vi "STATION.vi"(6 "station":T4, 8 "error_in":errorcluster, 11 "all_config_info":T1) -> (0 "error_out":errorcluster)   [LabVIEW 2020]
uses:
  station.ctl
  ini/typedef/PROXY_all_config_info.ctl
  ini/typedef/PROXY_main_ini_file.ctl
  queues/typedef/PROXY_queue_refnums.ctl
  queues/typedef/STATION_queue_element.ctl
  ST_SQL_sequence_state.ctl
  ST_TCP_sequence_state.ctl
  FGV/DIAGNOSTICS_records_display/FGV_PROXY_DIAGNOSTICS_records_display.ctl
  MAIN/DIAGNOSTICS/PROXY_SQL_connection_status.ctl
  FGV/SQL_part_ID_buffer/FGV_SQL_part_ID_buffer.ctl
  FGV/SQL_pinion_ID_buffer/FGV_SQL_pinion_ID_buffer.ctl
  FGV/connection_references/FGV_PROXY_connection_references.ctl
  FGV/DIAGNOSTICS_message_history_buffer/FGV_PROXY_DIAGNOSTICS_message_history_buffer.ctl
  FGV/error_buffer/FGV_PROXY_error_buffer.ctl
  <vilib>/addons/database/Connection.llb/Conn ObjectReference.ctl
  _misc/PLC_connection_status.ctl
  <vilib>/addons/database/Connection.llb/DB Tools Open Connec (String).vi
  _misc/byte_array_parser/to_U16.vi
  _misc/byte_array_parser/to_string.vi
  _misc/byte_array_parser/to_U8.vi
  _misc/AULocalize/SubVIs/Get Localized Phrase Compact Interface 0D.vi
  <vilib>/addons/database/NI_Database_API.lvlib
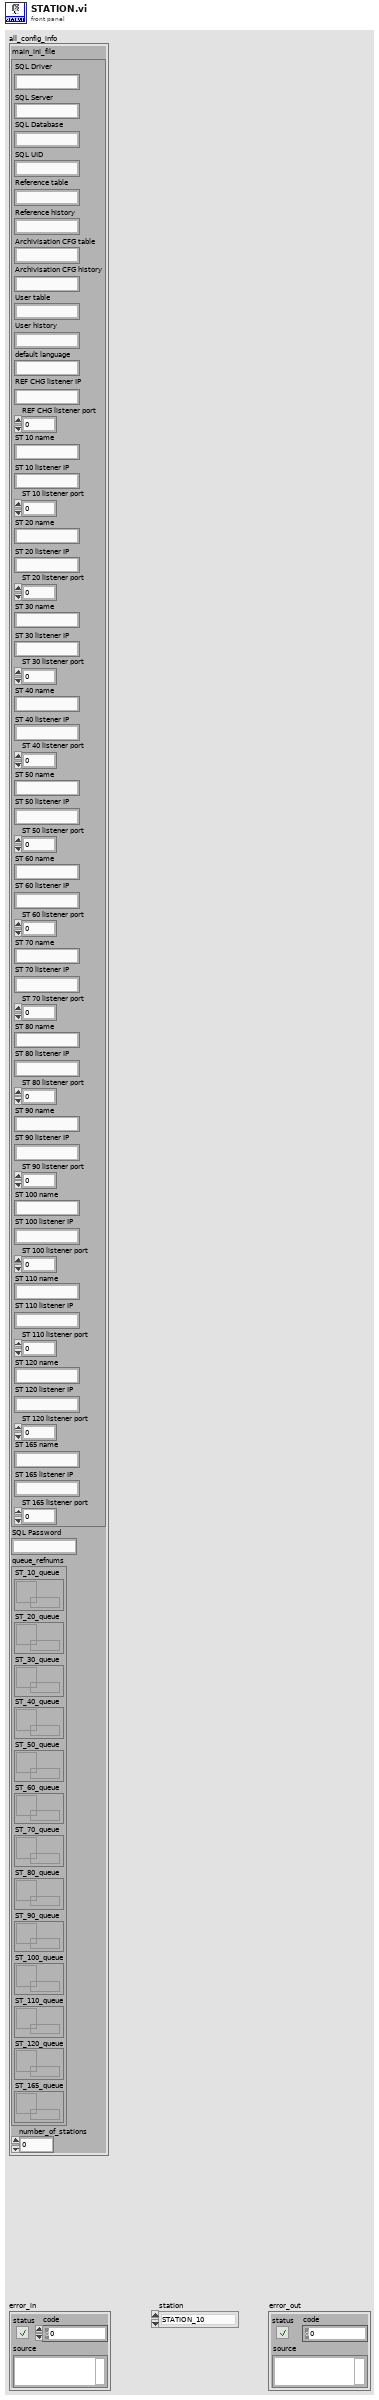
[diagram p1: front panel]
types:
  T1 = typedef "PROXY_all_config_info.ctl" = cluster{"main_ini_file":T2, "SQL Password":string, "queue_refnums":T3, "number_of_stations":i32}
  T2 = typedef "PROXY_main_ini_file.ctl" = cluster{"SQL Driver":string, "SQL Server":string, "SQL Database":string, "SQL UID":string, "Reference table":string, "Reference history":string, "Archivisation CFG table":string, "Archivisation CFG history":string, "User table":string, "User history":string, "default language":string, "REF CHG listener IP":string, "REF CHG listener port":u16, "ST 10 name":string, "ST 10 listener IP":string, "ST 10 listener port":u16, "ST 20 name":string, "ST 20 listener IP":string, "ST 20 listener port":u16, "ST 30 name":string, "ST 30 listener IP":string, "ST 30 listener port":u16, "ST 40 name":string, "ST 40 listener IP":string, "ST 40 listener port":u16, "ST 50 name":string, "ST 50 listener IP":string, "ST 50 listener port":u16, "ST 60 name":string, "ST 60 listener IP":string, "ST 60 listener port":u16, "ST 70 name":string, "ST 70 listener IP":string, "ST 70 listener port":u16, "ST 80 name":string, "ST 80 listener IP":string, "ST 80 listener port":u16, "ST 90 name":string, "ST 90 listener IP":string, "ST 90 listener port":u16, "ST 100 name":string, "ST 100 listener IP":string, "ST 100 listener port":u16, "ST 110 name":string, "ST 110 listener IP":string, "ST 110 listener port":u16, "ST 120 name":string, "ST 120 listener IP":string, "ST 120 listener port":u16, "ST 165 name":string, "ST 165 listener IP":string, "ST 165 listener port":u16}
  T3 = typedef "PROXY_queue_refnums.ctl" = cluster{"ST_10_queue":refnum<queue>, "ST_20_queue":refnum<queue>, "ST_30_queue":refnum<queue>, "ST_40_queue":refnum<queue>, "ST_50_queue":refnum<queue>, "ST_60_queue":refnum<queue>, "ST_70_queue":refnum<queue>, "ST_80_queue":refnum<queue>, "ST_90_queue":refnum<queue>, "ST_100_queue":refnum<queue>, "ST_110_queue":refnum<queue>, "ST_120_queue":refnum<queue>, "ST_165_queue":refnum<queue>}
  T4 = typedef "station.ctl" = enum16{"STATION_10", "STATION_20", "STATION_30", "STATION_40", "STATION_50", "STATION_60", "STATION_70", "STATION_80", "STATION_90", "STATION_100", "STATION_110", "STATION_120", "STATION_165", "MAIN"}
  T5 = typedef "ST_TCP_sequence_state.ctl" = enum16{"initialize", "wait_for_connection", "handle_message", "error", "stop"}
  T6 = typedef "ST_SQL_sequence_state.ctl" = enum16{"initialize", "get_next_state", "send_to_SQL", "send_to_PLC", "error", "stop"}
  T7 = typedef "FGV_PROXY_connection_references.ctl" = enum16{"initialize", "set_listener_ID", "set_connection_ID", "get", "KILL_ALL_CONNECTIONS", "killed?"}
  T8 = typedef "PLC_connection_status.ctl" = enum16{"Connected", "Waiting", "Error", "-"}
  T9 = typedef "FGV_PROXY_DIAGNOSTICS_records_display.ctl" = enum16{"initialize", "set_PLC_IP", "set_PLC_Port", "set_PLC_connection_status", "set_SQL_connection_status", "get_all_info"}
  T10 = enum16{"Standard", "Buffered", "CRLF", "Immediate"}
  T11 = typedef "STATION_queue_element.ctl" = cluster{"state":T6, "variable":variant}
  T12 = typedef "FGV_PROXY_DIAGNOSTICS_message_history_buffer.ctl" = enum16{"initialize", "add_TCP_PLC_to_PC", "add_TCP_PC_to_PLC", "add_SQL_PC_to_DB", "add_SQL_transaction", "add_SQL_DB_to_PC", "get_station", "get_all", "clear_station", "clear_all", "save_log"}
  T13 = typedef "FGV_PROXY_error_buffer.ctl" = enum16{"initialize", "clear", "display", "get_status"}
  T14 = typedef "PROXY_SQL_connection_status.ctl" = enum16{"Connected", "Waiting", "Error", "-"}
  T15 = typedef "FGV_SQL_part_ID_buffer.ctl" = enum16{"initialize", "buffer_serial_ID", "get_ID_for_name"}
  T16 = typedef "FGV_SQL_pinion_ID_buffer.ctl" = enum16{"initialize", "buffer_pinion_ID", "buffer_pinion_ID_SQL", "get_ID_for_name"}
  T17 = typedef "NI_Database_API.lvlib/Conn ObjectReference.ctl" = refnum<k1>
  T18 = typedef "SQL_statuses.ctl" = enum16{"OK", "PART_IN_OPERATION", "PART_DOES_NOT_EXIST", "OPERATION_DOES_NOT_EXIST", "OPERATOR_DOES_NOT_EXIST", "PART_NOT_IN_OPERATION"}
  T19 = typedef "ST_results_info.ctl" = cluster{"INT_number":i32, "REAL_number":i32, "STRING_number":i32, "STRING_length":i32, "BATCH_number":i32, "BATCH_length":i32, "INT_array":i16[], "REAL_array":sgl[], "STRING_array":string[], "BATCH_array":string[]}
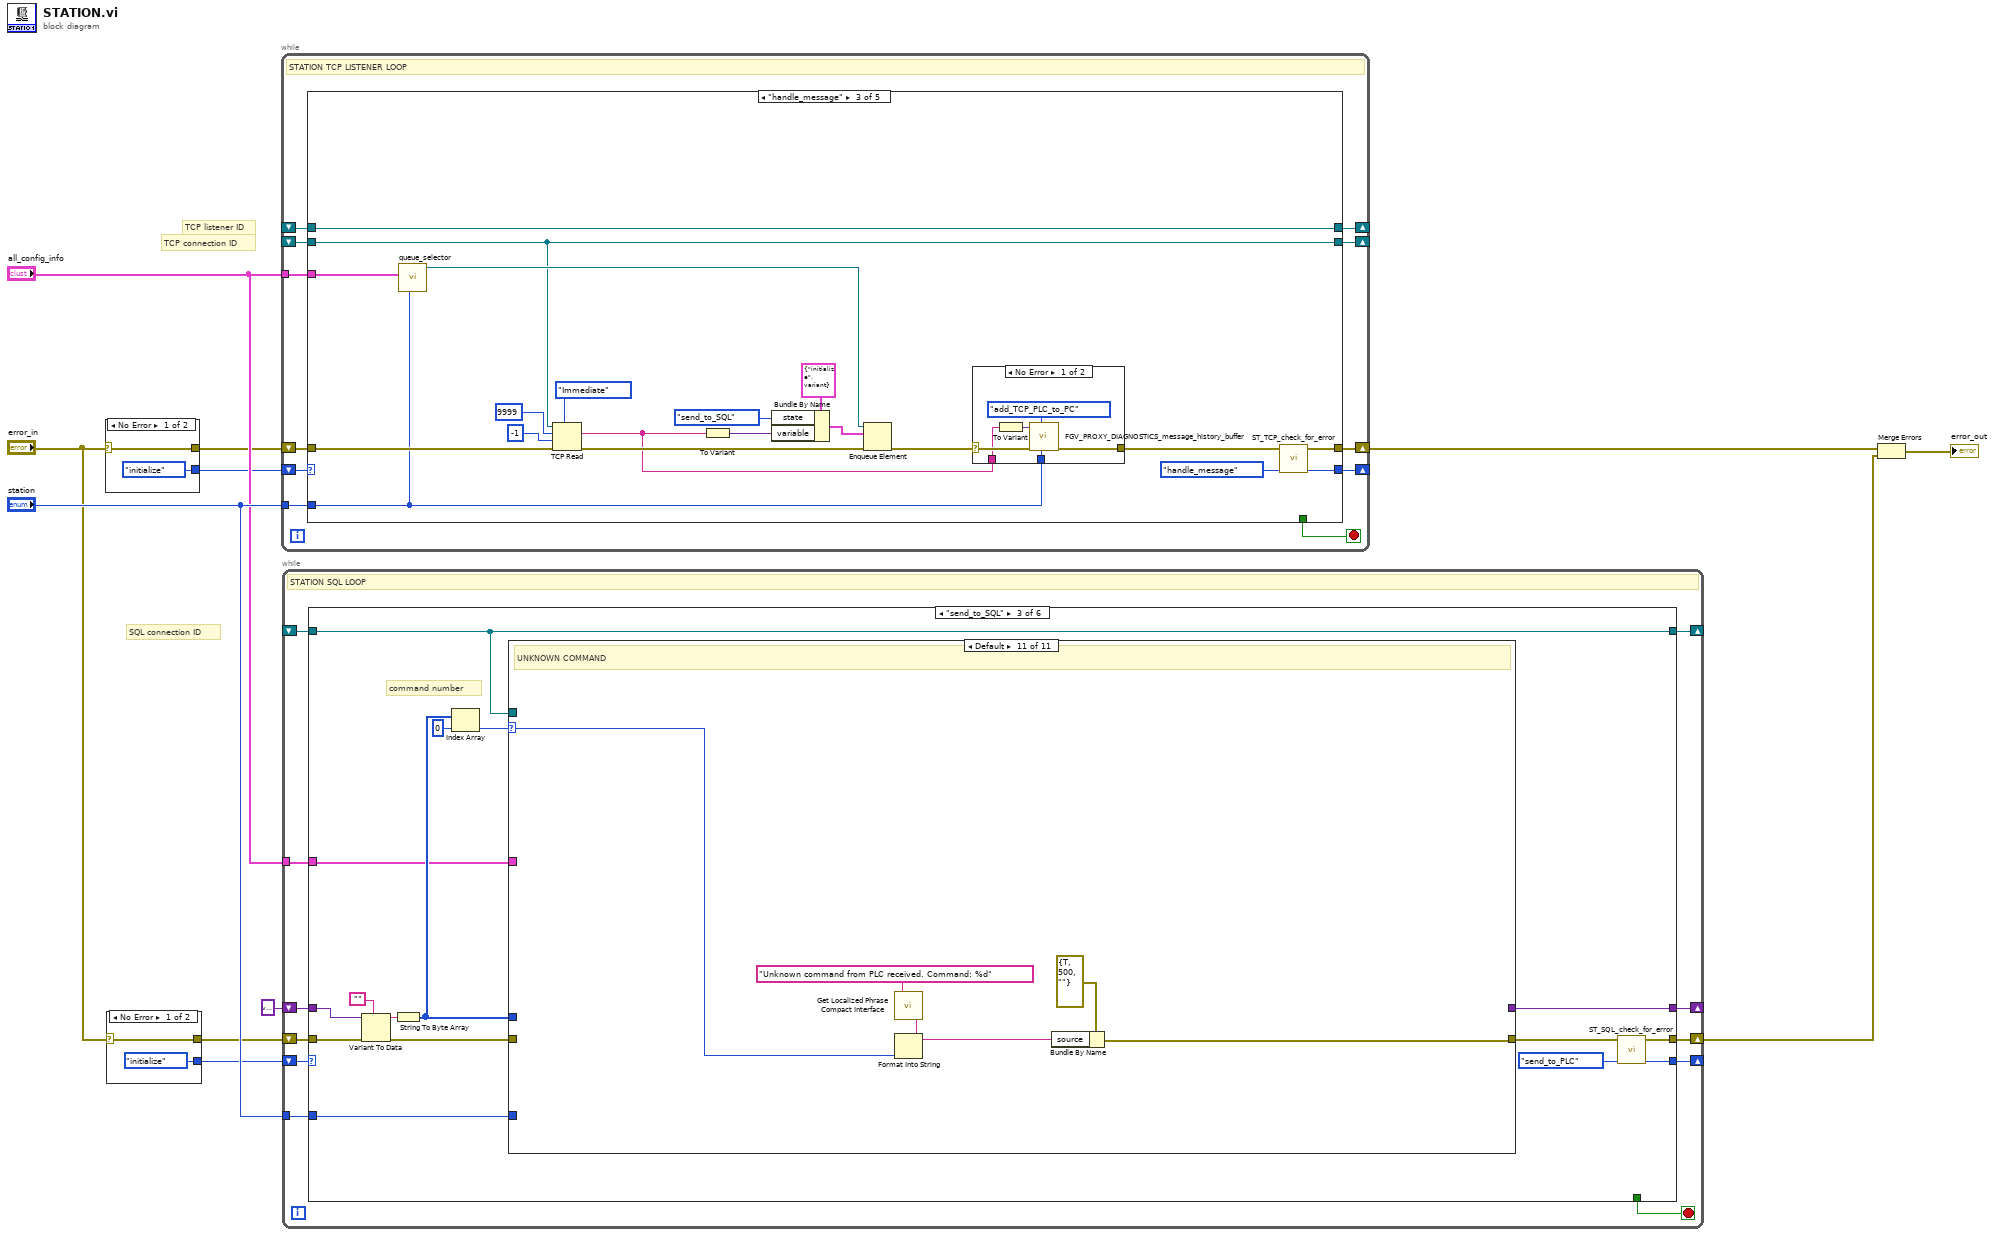
[diagram p0: block diagram]
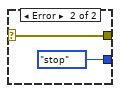
[diagram p2: hidden frame]
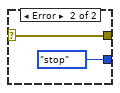
[diagram p3: hidden frame]
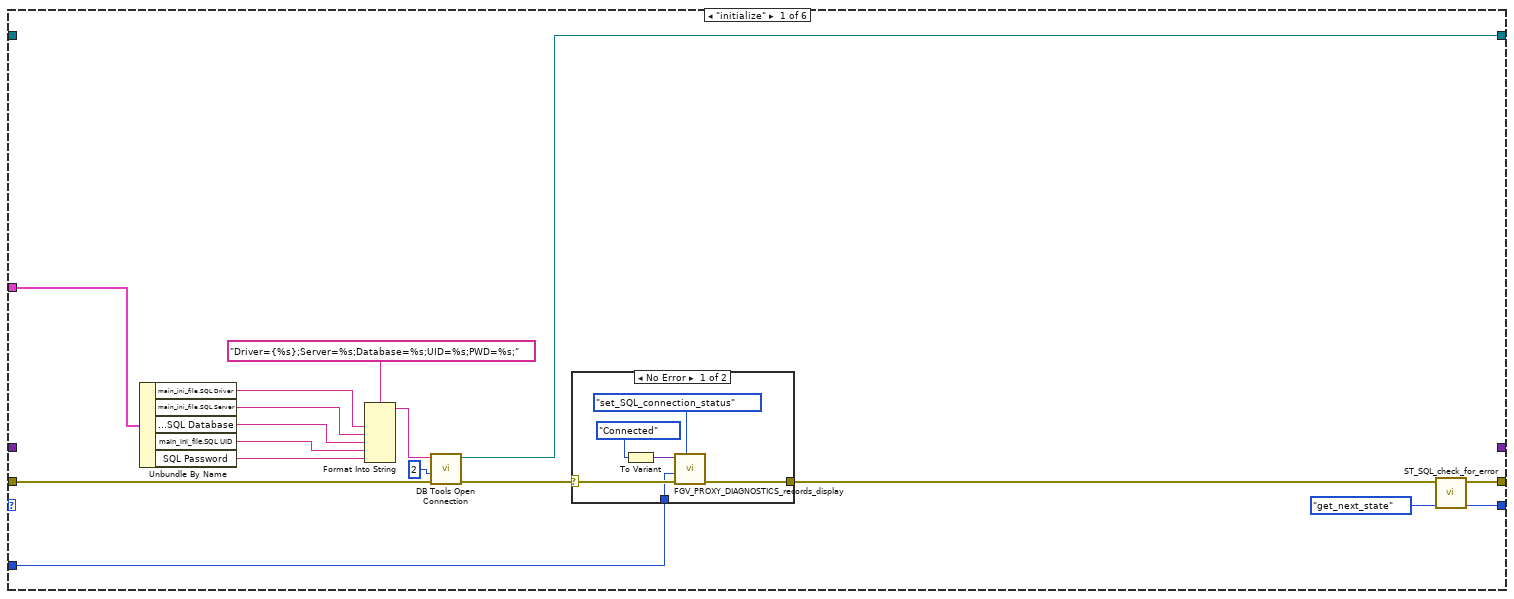
[diagram p4: hidden frame]
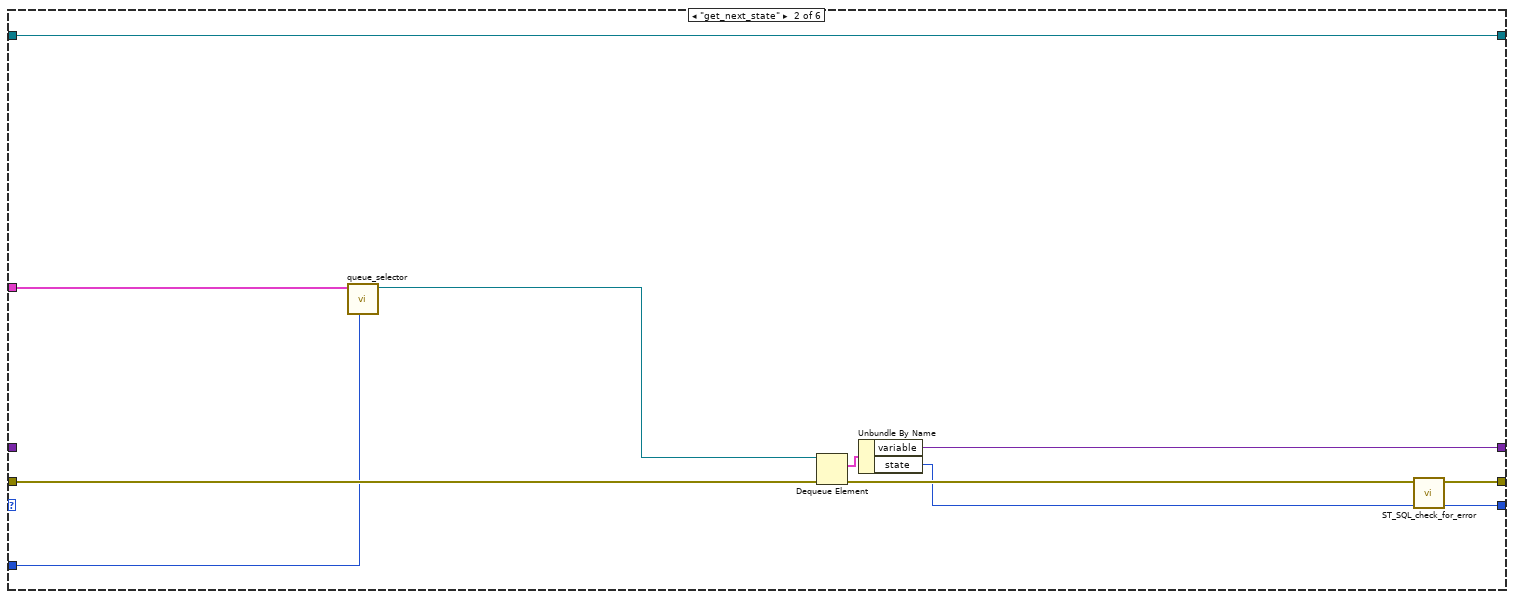
[diagram p6: hidden frame]
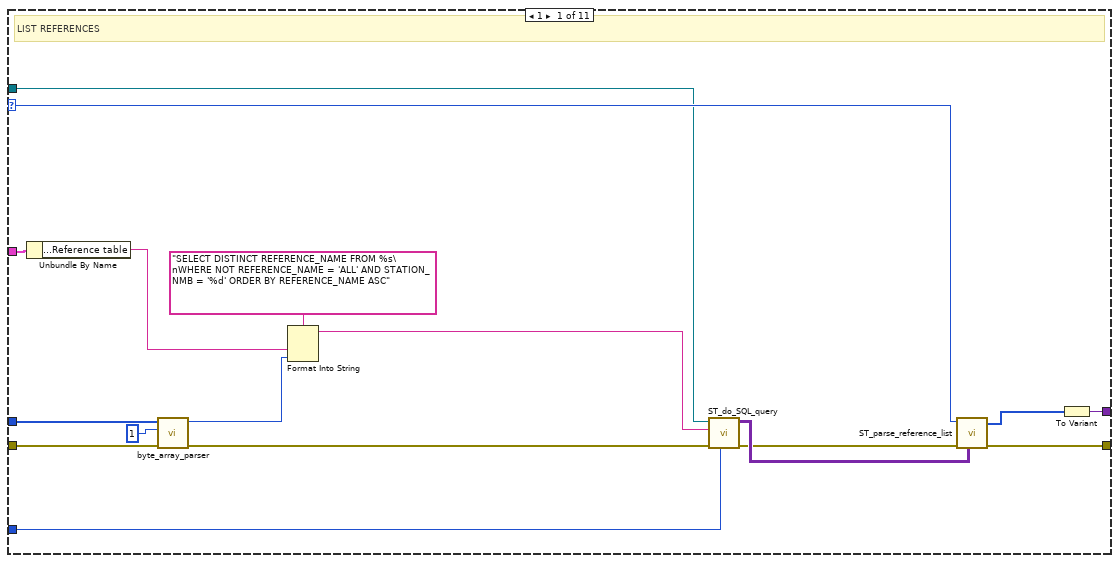
[diagram p7: hidden frame]
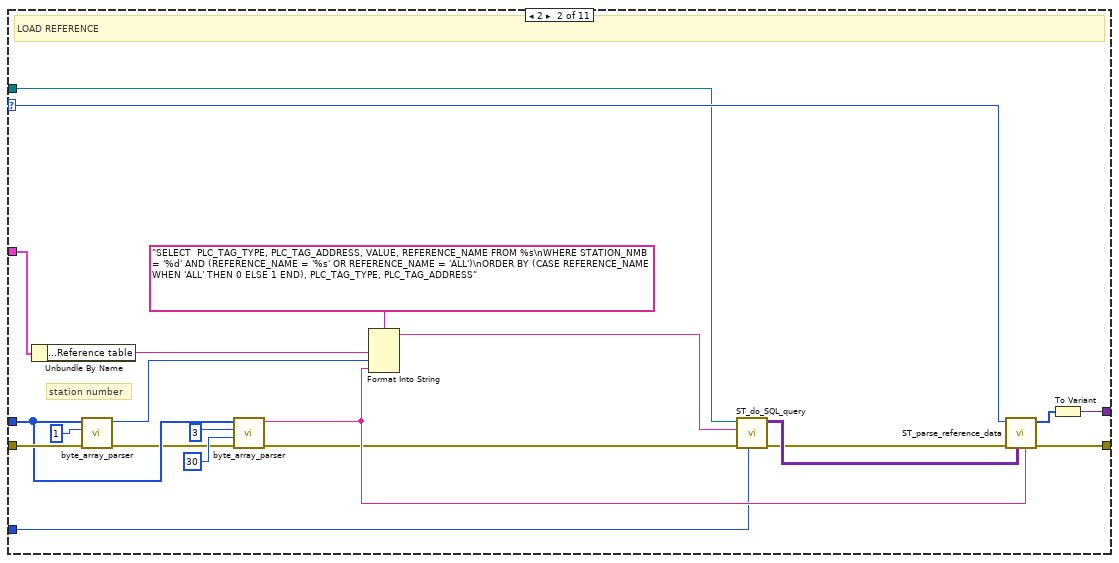
[diagram p8: hidden frame]
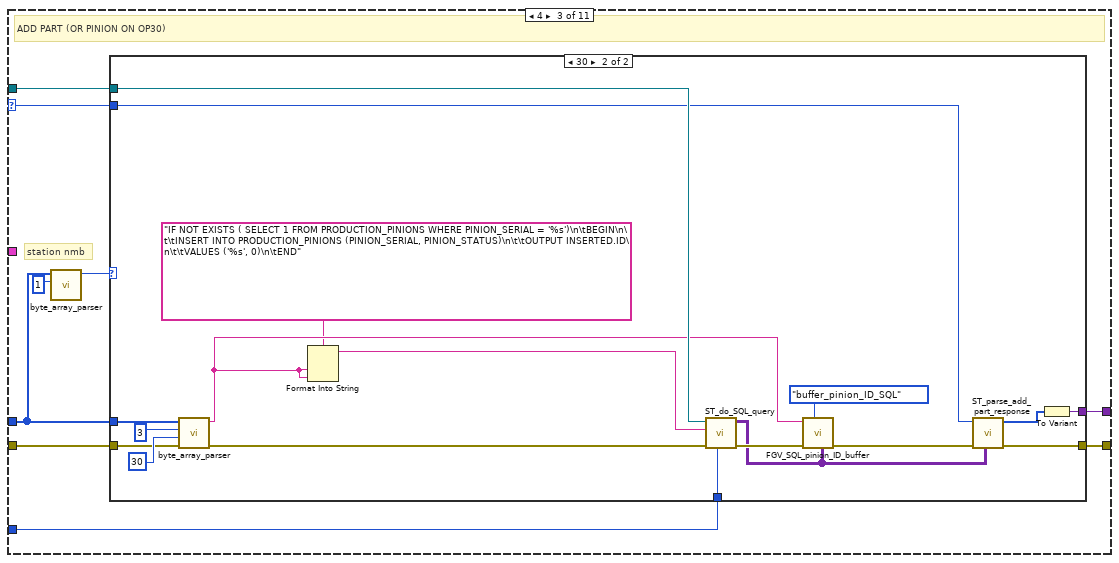
[diagram p9: hidden frame]
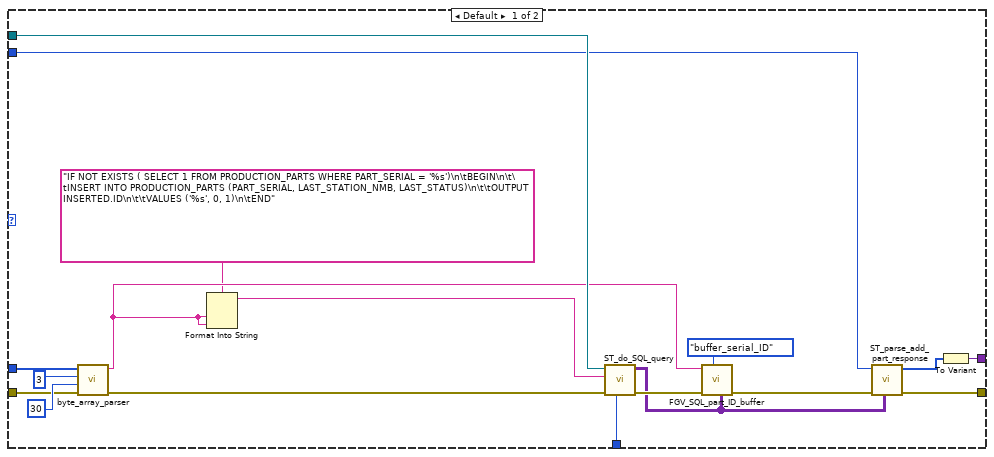
[diagram p10: hidden frame]
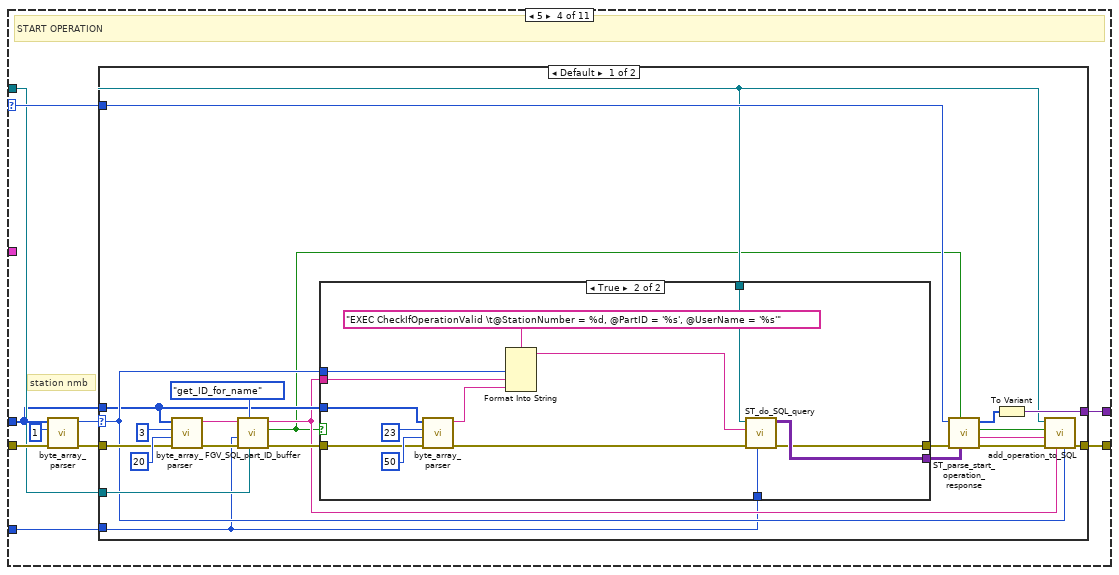
[diagram p11: hidden frame]
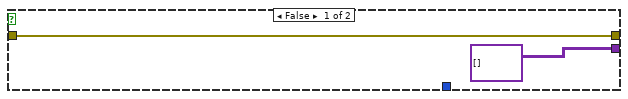
[diagram p12: hidden frame]
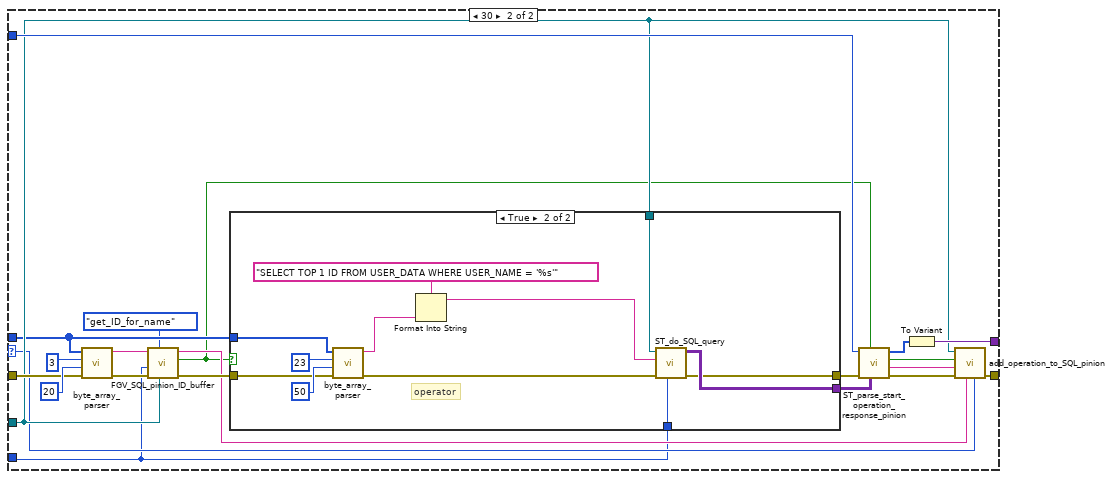
[diagram p13: hidden frame]
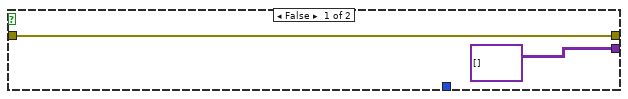
[diagram p14: hidden frame]
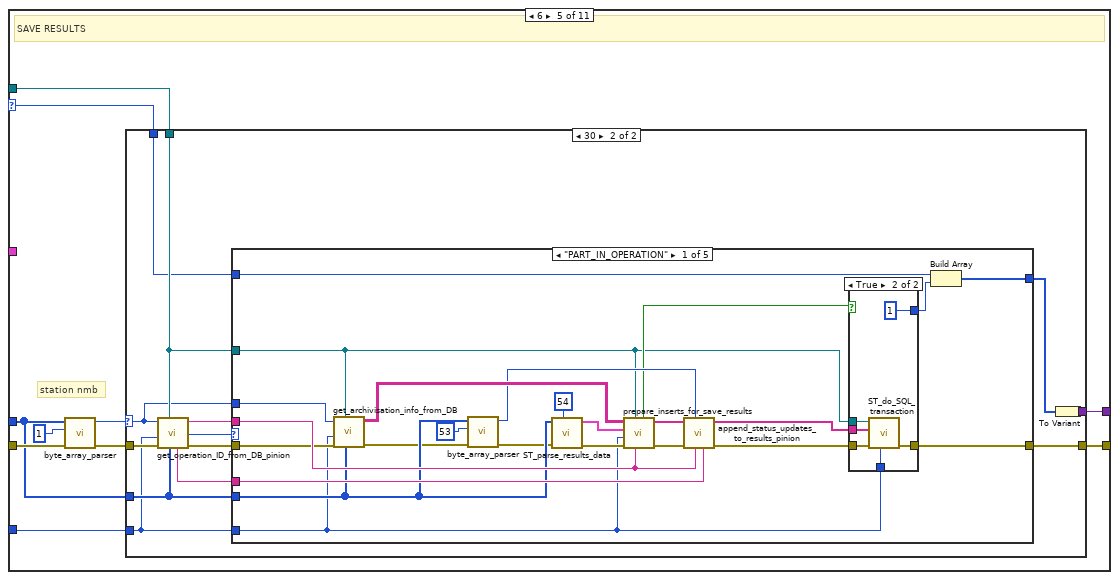
[diagram p15: hidden frame]
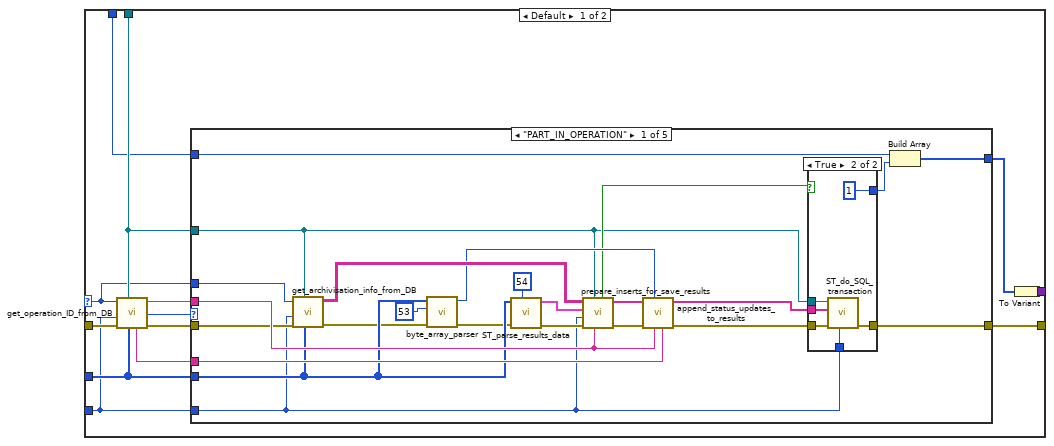
[diagram p16: hidden frame]
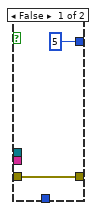
[diagram p17: hidden frame]
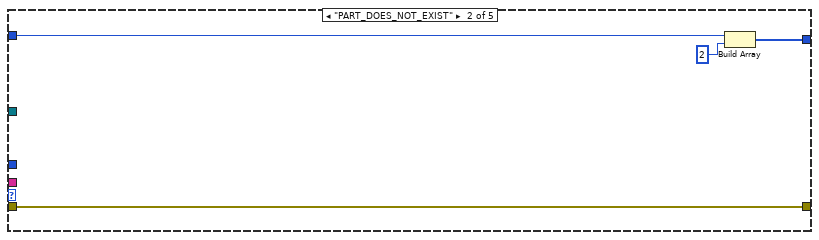
[diagram p18: hidden frame]
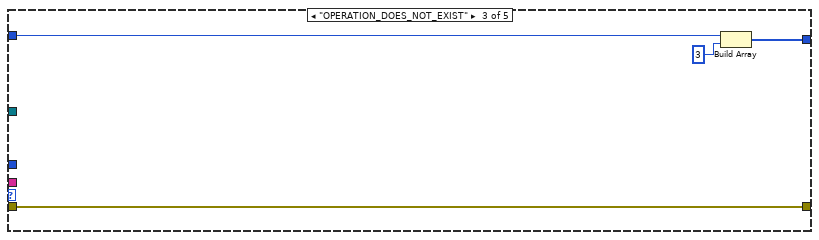
[diagram p19: hidden frame]
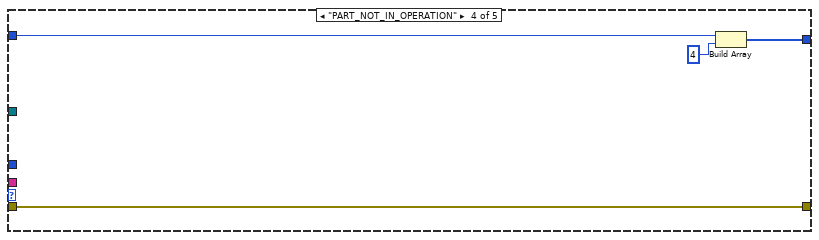
[diagram p20: hidden frame]
diagram:
  # "SQL connection ID"
  # "TCP connection ID"
  # "TCP listener ID"
  n1 = case shown="No Error" "error_in" {
    selector: "error_in" -> [w12 w14]
    tunnel: [ST_TCP_sequence_state."initialize" ("PLC_TCP_1_loop_states") ST_TCP_sequence_state."stop" ("PLC_TCP_1_loop_states")] -> w5
    tunnel: [w12 w14] -> w1
    frame No Error {
    }
    frame Error {
    }
  }
  n2 = case shown="No Error" "error_in" {
    selector: "error_in" -> [w16 w18]
    tunnel: [ST_SQL_sequence_state."initialize" ("PLC_TCP_1_loop_states") ST_SQL_sequence_state."stop" ("PLC_TCP_1_loop_states")] -> w4
    tunnel: [w16 w18] -> w2
    frame No Error {
    }
    frame Error {
    }
  }
  n3 = while {
    shift-right: [w23] -> _
    shift-left: w5 -> [w30]
    shift-right: [w22] -> w6
    shift-left: w1 -> [w28]
    shift-right: [w27] -> _
    shift-left: _ -> [w26]
    tunnel: "all_config_info" -> [w25]
    tunnel: "station" -> [w24]
    shift-right: [w21] -> _
    shift-left: _ -> [w20]
    stop <- w29 stop-if-true
    # "STATION TCP LISTENER LOOP"
    n4 = case shown="\"handle_message\"" w30 {
      tunnel: [_ _ _ _ TRUE] -> w29
      tunnel: w28 -> [_ w46 w78 w97 w104]
      tunnel: [w35 w58 w77 w101 w106] -> w22
      tunnel: [w42 w55 w81 w96 w103] -> w27
      tunnel: w26 -> [_ w55 w81 w96 _]
      tunnel: w25 -> [w38 _ w74 _ w109]
      tunnel: w24 -> [w32 w44 w65 w89 w108]
      tunnel: [w34 w56 w76 w98 ST_TCP_sequence_state."stop" ("PLC_TCP_loop_state_in")] -> w23
      tunnel: [refnum<k5> refnum ("connection ID") w54 w67 w95 w103] -> w21
      tunnel: w20 -> [_ _ w67 w95 _]
      frame "initialize" {
        n5 = call "listener_parameters_selector.vi"("stations"=w32, "all_config_info_out"=w38) -> ("listener port"=w40:u16, "listener IP"=w39:string)  [unwired: 8 in]
        n6 = String To IP(1:w39) -> (0:w41:u32)
        n7 = TCP Create Listener(7:w41, 10:w40) -> (0:w37:errorcluster, 3:w42:refnum<k5>)  [unwired: 3 in, 1 out]
        n8 = call "FGV_PROXY_connection_references.vi"("station"=w32, "options"=FGV_PROXY_connection_references."set_listener_ID", "error_in"=w37, "reference_in"=w42) -> ("error_out"=w36:errorcluster)  [unwired: 4 in, 3 out]
        n9 = call "ST_TCP_check_for_error.vi"("PLC_TCP_loop_state_in"=ST_TCP_sequence_state."wait_for_connection", "error_in"=w36) -> ("PLC_TCP_loop_state_out"=w34:T5, "error_out"=w35:errorcluster)  [unwired: 8 in]
      }
      frame "wait_for_connection" {
        n10 = To Variant(anything=PLC_connection_status."Waiting" ("connection_status")) -> (Variant=w47:variant)
        n11 = call "FGV_PROXY_DIAGNOSTICS_records_display.vi"("options"=FGV_PROXY_DIAGNOSTICS_records_display."set_PLC_connection_status", "error_in"=w46, "station"=w44, "input"=w47) -> ("error_out"=w45:errorcluster)  [unwired: 6 in, 1 out]
        n12 = TCP Wait On Listener(8:w45, 10:FALSE ("resolve remote address (T)"), 11:w55) -> (0:w52:errorcluster, 1:w50:u16, 2:w51:string, 4:w54:refnum<k5>)  [unwired: 1 in, 1 out]
        n13 = call "PROXY_set_IP_and_port_after_connection_established.vi"("station"=w44, "error_in"=w52, "PLC_port"=w50, "PLC_IP"=w51) -> ("error_out"=w53:errorcluster)  [unwired: 7 in]
        n14 = call "FGV_PROXY_connection_references.vi"("station"=w44, "options"=FGV_PROXY_connection_references."set_connection_ID", "error_in"=w53, "reference_in"=w54) -> ("error_out"=w59:errorcluster)  [unwired: 4 in, 3 out]
        n15 = call "ST_TCP_check_for_error.vi"("PLC_TCP_loop_state_in"=ST_TCP_sequence_state."handle_message" ("PLC_TCP_1_loop_states"), "error_in"=w59) -> ("PLC_TCP_loop_state_out"=w56:T5, "error_out"=w58:errorcluster)  [unwired: 8 in]
      }
      frame "handle_message" {
        n16 = call "queue_selector.vi"("station"=w65, "all_config_info_in"=w74) -> ("queue_out"=w73:refnum<queue>)  [unwired: 9 in]
        n17 = TCP Read(connection ID=w67, bytes to read=9999, error in (no error)=w78, 7:T10."Immediate" ("mode (standard)"), 9:-1 ("timeout ms (25000)")) -> (data out=w62:string, error out=w69:errorcluster)  [unwired: 1 out]
        n18 = To Variant(anything=w62) -> (Variant=w68:variant)
        n19 = Bundle By Name(cluster=T11 {"state"=enum."initialize", "variable"=variant} ("element"), "state"=ST_SQL_sequence_state."send_to_SQL", "variable"=w68) -> (w71:T11)
        n20 = Enqueue Element(queue=w73, element=w71, error in (no error)=w69) -> (error out=w64:errorcluster)  [unwired: 1 in, 2 out]
        n21 = case shown="No Error" w64 {
          selector: w64 -> [w85 w88]
          tunnel: w65 -> [w86 _]
          tunnel: [w84 w88] -> w63
          tunnel: w62 -> [w83 _]
          frame No Error {
            n22 = To Variant(anything=w83) -> (Variant=w82:variant)
            n23 = call "FGV_PROXY_DIAGNOSTICS_message_history_buffer.vi"("station"=w86, "options"=FGV_PROXY_DIAGNOSTICS_message_history_buffer."add_TCP_PLC_to_PC", "error_in"=w85, "input"=w82) -> ("error_out"=w84:errorcluster)  [unwired: 6 in, 1 out]
          }
          frame Error {
          }
        }
        n24 = call "ST_TCP_check_for_error.vi"("PLC_TCP_loop_state_in"=ST_TCP_sequence_state."handle_message", "error_in"=w63) -> ("PLC_TCP_loop_state_out"=w76:T5, "error_out"=w77:errorcluster)  [unwired: 8 in]
      }
      frame "error" {
        # "don't go to initialize, because listener should be created only once\nmaybe move it before loop later, don't know yet"
        n25 = call "FGV_PROXY_error_buffer.vi"("station"=w89, "option"=FGV_PROXY_error_buffer."display", "error_in"=w97) -> ("error_out"=w91:errorcluster)  [unwired: 7 in, 1 out]
        n26 = To Variant(anything=PLC_connection_status."Error" ("connection_status")) -> (Variant=w92:variant)
        n27 = call "FGV_PROXY_DIAGNOSTICS_records_display.vi"("options"=FGV_PROXY_DIAGNOSTICS_records_display."set_PLC_connection_status", "error_in"=w91, "station"=w89, "input"=w92) -> ("error_out"=w90:errorcluster)  [unwired: 6 in, 1 out]
        n28 = call "ST_TCP_check_for_error.vi"("PLC_TCP_loop_state_in"=ST_TCP_sequence_state."wait_for_connection", "error_in"=w90) -> ("PLC_TCP_loop_state_out"=w98:T5, "error_out"=w101:errorcluster)  [unwired: 8 in]
        n29 = call "wait_on_initialization.vi"("state"=w98) -> ()  [unwired: 11 in]
      }
      frame "stop" {
        w103 = refnum<k5> refnum ("connection ID")
        n30 = call <vilib>:"Clear Errors.vi"("error in (no error)"=w104) -> ("error out"=w107:errorcluster)  [unwired: 5 in, 1 out]
        n31 = call "queue_selector.vi"("station"=w108, "all_config_info_in"=w109) -> ("queue_out"=w105:refnum<queue>)  [unwired: 9 in]
        n32 = Enqueue Element(queue=w105, element=T11 {"state"=enum."stop", "variable"=variant}, error in (no error)=w107) -> (error out=w106:errorcluster)  [unwired: 1 in, 2 out]
      }
    }
  }
  n33 = while {
    shift-right: [w116] -> _
    shift-left: w4 -> [w122]
    shift-right: [w119] -> w7
    shift-left: w2 -> [w120]
    tunnel: "all_config_info" -> [w118]
    tunnel: "station" -> [w117]
    shift-right: [w115] -> _
    shift-left: variant ("variable") -> [w114]
    shift-right: [w113] -> _
    shift-left: _ -> [w112]
    stop <- w121 stop-if-true
    # "STATION SQL LOOP"
    n34 = case shown="\"send_to_SQL\"" w122 {
      tunnel: [_ _ _ _ _ TRUE] -> w121
      tunnel: w120 -> [w136 w155 w170 w668 w688 w699]
      tunnel: [w139 w157 w173 w676 w697 w703] -> w119
      tunnel: w118 -> [w133 w149 w161 _ _ _]
      tunnel: w117 -> [w123 w153 w158 w666 w684 _]
      tunnel: [w137 w156 w171 w675 w694 ST_SQL_sequence_state."stop" ("PLC_MAIN_loop_state_out")] -> w116
      tunnel: [_ w148 w162 _ _ _] -> w115
      tunnel: w114 -> [_ _ w169 w669 _ _]
      tunnel: [w127 w152 w163 w670 w690 w700] -> w113
      tunnel: w112 -> [_ w152 w163 w670 w693 w701]
      frame "initialize" {
        n35 = Unbundle By Name(w133) -> ("main_ini_file.SQL Driver"=w132:string, "main_ini_file.SQL Server"=w131:string, "main_ini_file.SQL Database"=w130:string, "main_ini_file.SQL UID"=w129:string, "SQL Password"=w128:string)
        n36 = Format Into String(format string="Driver={%s};Server=%s;Database=%s;UID=%s;PWD=%s;", w132, w131, w130, w129, w128) -> (resulting string=w135:string)  [unwired: 2 in, 1 out]
        n37 = call-poly <vilib>:"DB Tools Open Connection.vi"("error in (no error)"=w136, "connection timeout (15)"=2, "connection information"=w135) -> ("error out"=w125:errorcluster, "connection reference"=w127:T17)  [unwired: 5 in]
        n38 = case shown="No Error" w125 {
          selector: w125 -> [w142 w146]
          tunnel: [w141 w146] -> w124
          tunnel: w123 -> [w140 _]
          frame No Error {
            n39 = To Variant(anything=PROXY_SQL_connection_status."Connected" ("SQL_connection_status")) -> (Variant=w144:variant)
            n40 = call "FGV_PROXY_DIAGNOSTICS_records_display.vi"("options"=FGV_PROXY_DIAGNOSTICS_records_display."set_SQL_connection_status", "error_in"=w142, "station"=w140, "input"=w144) -> ("error_out"=w141:errorcluster)  [unwired: 6 in, 1 out]
          }
          frame Error {
          }
        }
        n41 = call "ST_SQL_check_for_error.vi"("ST_SQL_loop_state_in"=ST_SQL_sequence_state."get_next_state" ("ST_MAIN_sequence_state"), "error_in"=w124) -> ("ST_SQL_loop_state_out"=w137:T6, "error_out"=w139:errorcluster)  [unwired: 8 in]
      }
      frame "get_next_state" {
        n42 = call "queue_selector.vi"("station"=w153, "all_config_info_in"=w149) -> ("queue_out"=w147:refnum<queue>)  [unwired: 9 in]
        n43 = Dequeue Element(queue=w147, error in (no error)=w155) -> (element=w151:T11, error out=w154:errorcluster)  [unwired: 1 in, 2 out]
        n44 = Unbundle By Name(w151) -> ("variable"=w148:variant, "state"=w150:T6)
        n45 = call "ST_SQL_check_for_error.vi"("ST_SQL_loop_state_in"=w150, "error_in"=w154) -> ("ST_SQL_loop_state_out"=w156:T6, "error_out"=w157:errorcluster)  [unwired: 8 in]
      }
      frame "send_to_SQL" {
        # "command number"
        n46 = Variant To Data(error in=w170, type="", Variant=w169) -> (data=w167:string, error out=w160:errorcluster)
        n47 = String To Byte Array(string=w167) -> (unsigned byte array=w164:u8[])
        n48 = Index Array(array=w164, index=0) -> (element=w159:u8)
        n49 = case shown="Default" w159 {
          selector: w159 -> [w182 w201 w216 w262 w346 w483 w503 w541 w549 w614 w658]
          tunnel: w160 -> [w185 w210 w218 w264 w349 w490 w496 w532 w564 w612 _]
          tunnel: [w187 w198 w217 w260 w348 w480 w500 w542 w550 w615 w656] -> w165
          tunnel: w164 -> [w184 w204 w213 w258 w342 w486 w495 w529 w552 w611 _]
          tunnel: w163 -> [w180 w199 w220 w261 w347 w481 w502 w545 w553 w602 _]
          tunnel: [w188 w206 w219 w266 w345 w488 w512 w524 w548 w609 _] -> w162
          tunnel: w161 -> [w177 w205 _ _ _ w487 _ _ _ _ _]
          tunnel: w158 -> [w175 w192 w215 w257 w341 w471 w492 w536 w546 w600 _]
          frame 1 {
            # "LIST REFERENCES"
            n50 = Unbundle By Name(w177) -> ("main_ini_file.Reference table"=w189:string)
            n51 = call-poly "byte_array_parser.vi"("error_in"=w185, "variable_start_index"=1, "byte_array"=w184) -> ("error_out"=w176:errorcluster, "U16"=w183:u16)  [unwired: 7 in]
            n52 = Format Into String(format string="SELECT DISTINCT REFERENCE_NAME FROM %s\nWHERE NOT REFERENCE_NAME = 'ALL' AND STATION_NMB = '%d' ORDER BY REFERENCE_NAME ASC", w189, w183) -> (resulting string=w179:string)  [unwired: 2 in, 1 out]
            n53 = call "ST_do_SQL_query.vi"("station"=w175, "error_in"=w176, "SQL_query"=w179, "SQL_connection_reference"=w180) -> ("error_out"=w174:errorcluster, "recordset_out"=w178:variant[][])  [unwired: 6 in]
            n54 = call "ST_parse_reference_list.vi"("recordset_data"=w178, "error_in"=w174, "command_nmb"=w182) -> ("error_out"=w187:errorcluster, "reference_data_to_PLC"=w181:u8[])  [unwired: 7 in]
            n55 = To Variant(anything=w181) -> (Variant=w188:variant)
          }
          frame 2 {
            # "station number"
            # "LOAD REFERENCE"
            n56 = Unbundle By Name(w205) -> ("main_ini_file.Reference table"=w208:string)
            n57 = call-poly "byte_array_parser.vi"("error_in"=w210, "variable_start_index"=1, "byte_array"=w204) -> ("error_out"=w196:errorcluster, "U16"=w207:u16)  [unwired: 7 in]
            n58 = call-poly "byte_array_parser.vi"("error_in"=w196, "string_length"=30, "variable_start_index"=3, "byte_array"=w204) -> ("error_out"=w193:errorcluster, "string"=w194:string)  [unwired: 6 in]
            n59 = Format Into String(format string="SELECT  PLC_TAG_TYPE, PLC_TAG_ADDRESS, VALUE, REFERENCE_NAME FROM %s\nWHERE STATION_NMB = '%d' AND (REFERENCE_NAME = '%s' OR REFERENCE_NAME = 'ALL')\nORDER BY (CASE REFERENCE_NAME WHEN 'ALL' THEN 0 ELSE 1 END), PLC_TAG_TYPE, PLC_TAG_ADDRESS", w208, w207, w194) -> (resulting string=w195:string)  [unwired: 2 in, 1 out]
            n60 = call "ST_do_SQL_query.vi"("station"=w192, "error_in"=w193, "SQL_query"=w195, "SQL_connection_reference"=w199) -> ("error_out"=w191:errorcluster, "recordset_out"=w197:variant[][])  [unwired: 6 in]
            n61 = call "ST_parse_reference_data.vi"("reference_name"=w194, "recordset_data"=w197, "error_in"=w191, "command_nmb"=w201) -> ("error_out"=w198:errorcluster, "reference_data_to_PLC"=w200:u8[])  [unwired: 6 in]
            n62 = To Variant(anything=w200) -> (Variant=w206:variant)
          }
          frame 4 {
            # "station nmb"
            # "ADD PART (OR PINION ON OP30)"
            n63 = call-poly "byte_array_parser.vi"("variable_start_index"=1, "byte_array"=w213) -> ("U16"=w212:u16)  [unwired: 8 in, 1 out]
            n64 = case shown="30" w212 {
              tunnel: w220 -> [w238 w256]
              tunnel: [w237 w255] -> w219
              tunnel: w213 -> [w236 w254]
              tunnel: w218 -> [w231 w250]
              tunnel: [w230 w249] -> w217
              tunnel: w216 -> [w228 w247]
              tunnel: w215 -> [w221 w241]
              frame Default {
                n65 = call-poly "byte_array_parser.vi"("error_in"=w231, "string_length"=30, "variable_start_index"=3, "byte_array"=w236) -> ("error_out"=w223:errorcluster, "string"=w227:string)  [unwired: 6 in]
                n66 = Format Into String(format string="IF NOT EXISTS ( SELECT 1 FROM PRODUCTION_PARTS WHERE PART_SERIAL = '%s')\n\tBEGIN\n\t\tINSERT INTO PRODUCTION_PARTS (PART_SERIAL, LAST_STATION_NMB, LAST_STATUS)\n\t\tOUTPUT INSERTED.ID\n\t\tVALUES ('%s', 0, 1)\n\tEND", w227, w227) -> (resulting string=w224:string)  [unwired: 2 in, 1 out]
                n67 = call "ST_do_SQL_query.vi"("station"=w221, "error_in"=w223, "SQL_query"=w224, "SQL_connection_reference"=w238) -> ("error_out"=w233:errorcluster, "recordset_out"=w225:variant[][])  [unwired: 6 in]
                n68 = call "FGV_SQL_part_ID_buffer.vi"("recordset_in"=w225, "options"=FGV_SQL_part_ID_buffer."buffer_serial_ID", "error_in"=w233, "PART_SERIAL"=w227) -> ("error_out"=w222:errorcluster)  [unwired: 5 in, 2 out]
                n69 = call "ST_parse_add_part_response.vi"("recordset_in"=w225, "error_in"=w222, "command_nmb"=w228) -> ("error_out"=w230:errorcluster, "reference_data_to_PLC"=w229:u8[])  [unwired: 7 in]
                n70 = To Variant(anything=w229) -> (Variant=w237:variant)
              }
              frame 30 {
                n71 = call-poly "byte_array_parser.vi"("error_in"=w250, "string_length"=30, "variable_start_index"=3, "byte_array"=w254) -> ("error_out"=w243:errorcluster, "string"=w246:string)  [unwired: 6 in]
                n72 = Format Into String(format string="IF NOT EXISTS ( SELECT 1 FROM PRODUCTION_PINIONS WHERE PINION_SERIAL = '%s')\n\tBEGIN\n\t\tINSERT INTO PRODUCTION_PINIONS (PINION_SERIAL, PINION_STATUS)\n\t\tOUTPUT INSERTED.ID\n\t\tVALUES ('%s', 0)\n\tEND", w246, w246) -> (resulting string=w244:string)  [unwired: 2 in, 1 out]
                n73 = call "ST_do_SQL_query.vi"("station"=w241, "error_in"=w243, "SQL_query"=w244, "SQL_connection_reference"=w256) -> ("error_out"=w251:errorcluster, "recordset_out"=w239:variant[][])  [unwired: 6 in]
                n74 = call "FGV_SQL_pinion_ID_buffer.vi"("SQL_result"=w239, "options"=FGV_SQL_pinion_ID_buffer."buffer_pinion_ID_SQL", "error_in"=w251, "PINION_SERIAL"=w246) -> ("error_out"=w242:errorcluster)  [unwired: 5 in, 2 out]
                n75 = call "ST_parse_add_part_response.vi"("recordset_in"=w239, "error_in"=w242, "command_nmb"=w247) -> ("error_out"=w249:errorcluster, "reference_data_to_PLC"=w248:u8[])  [unwired: 7 in]
                n76 = To Variant(anything=w248) -> (Variant=w255:variant)
              }
            }
          }
          frame 5 {
            # "station nmb"
            # "START OPERATION"
            n77 = call-poly "byte_array_parser.vi"("error_in"=w264, "variable_start_index"=1, "byte_array"=w258) -> ("error_out"=w263:errorcluster, "U16"=w259:u16)  [unwired: 7 in]
            n78 = case shown="Default" w259 {
              selector: w259 -> [w273 w312]
              tunnel: [w288 w326] -> w266
              tunnel: w263 -> [w283 w322]
              tunnel: w262 -> [w278 w317]
              tunnel: w261 -> [w277 w316]
              tunnel: [w275 w314] -> w260
              tunnel: w258 -> [w271 w310]
              tunnel: w257 -> [w267 w306]
              frame Default {
                n79 = call-poly "byte_array_parser.vi"("error_in"=w283, "string_length"=20, "variable_start_index"=3, "byte_array"=w271) -> ("error_out"=w284:errorcluster, "string"=w282:string)  [unwired: 6 in]
                n80 = call "FGV_SQL_part_ID_buffer.vi"("connection reference"=w277, "options"=FGV_SQL_part_ID_buffer."get_ID_for_name", "error_in"=w284, "station"=w267, "PART_SERIAL"=w282) -> ("error_out"=w272:errorcluster, "Part exists?"=w268:bool, "ID_out"=w269:string)  [unwired: 4 in]
                n81 = case shown="True" w268 {
                  tunnel: w267 -> [_ w293]
                  tunnel: [w289 w291] -> w281
                  tunnel: [variant[][] [] ("recordset_out") w302] -> w280
                  tunnel: w277 -> [_ w301]
                  tunnel: w273 -> [_ w300]
                  tunnel: w269 -> [_ w299]
                  tunnel: w272 -> [w289 w296]
                  tunnel: w271 -> [_ w295]
                  frame False {
                  }
                  frame True {
                    n82 = call-poly "byte_array_parser.vi"("error_in"=w296, "string_length"=50, "variable_start_index"=23, "byte_array"=w295) -> ("error_out"=w292:errorcluster, "string"=w294:string)  [unwired: 6 in]
                    n83 = Format Into String(format string="EXEC CheckIfOperationValid \t@StationNumber = %d, @PartID = '%s', @UserName = '%s'", w300, w299, w294) -> (resulting string=w303:string)  [unwired: 2 in, 1 out]
                    n84 = call "ST_do_SQL_query.vi"("station"=w293, "error_in"=w292, "SQL_query"=w303, "SQL_connection_reference"=w301) -> ("error_out"=w291:errorcluster, "recordset_out"=w302:variant[][])  [unwired: 6 in]
                  }
                }
                n85 = call "ST_parse_start_operation_response.vi"("recordset_in"=w280, "Part exists?"=w268, "error_in"=w281, "command_nmb"=w278) -> ("error_out"=w276:errorcluster, "user_ID"=w270:string, "save_operation_to_SQL"=w274:bool, "reference_data_to_PLC"=w279:u8[])  [unwired: 4 in]
                n86 = To Variant(anything=w279) -> (Variant=w288:variant)
                n87 = call "add_operation_to_SQL.vi"("station_number"=w273, "part_ID"=w269, "error_in"=w276, "user_ID"=w270, "save_operation_to_SQL"=w274, "SQL_connection_reference"=w277) -> ("error_out"=w275:errorcluster)  [unwired: 5 in]
              }
              frame 30 {
                n88 = call-poly "byte_array_parser.vi"("error_in"=w322, "string_length"=20, "variable_start_index"=3, "byte_array"=w310) -> ("error_out"=w323:errorcluster, "string"=w321:string)  [unwired: 6 in]
                n89 = call "FGV_SQL_pinion_ID_buffer.vi"("connection reference"=w316, "options"=FGV_SQL_pinion_ID_buffer."get_ID_for_name", "error_in"=w323, "station"=w306, "PINION_SERIAL"=w321) -> ("error_out"=w311:errorcluster, "Pinion exists?"=w307:bool, "ID_out"=w308:string)  [unwired: 4 in]
                n90 = case shown="True" w307 {
                  tunnel: w306 -> [_ w331]
                  tunnel: [w327 w329] -> w320
                  tunnel: [variant[][] [] ("recordset_out") w338] -> w319
                  tunnel: w316 -> [_ w337]
                  tunnel: w311 -> [w327 w334]
                  tunnel: w310 -> [_ w333]
                  frame False {
                  }
                  frame True {
                    # "operator"
                    n91 = call-poly "byte_array_parser.vi"("error_in"=w334, "string_length"=50, "variable_start_index"=23, "byte_array"=w333) -> ("error_out"=w330:errorcluster, "string"=w332:string)  [unwired: 6 in]
                    n92 = Format Into String(format string="SELECT TOP 1 ID FROM USER_DATA WHERE USER_NAME = '%s'", w332) -> (resulting string=w339:string)  [unwired: 2 in, 1 out]
                    n93 = call "ST_do_SQL_query.vi"("station"=w331, "error_in"=w330, "SQL_query"=w339, "SQL_connection_reference"=w337) -> ("error_out"=w329:errorcluster, "recordset_out"=w338:variant[][])  [unwired: 6 in]
                  }
                }
                n94 = call "ST_parse_start_operation_response_pinion.vi"("recordset_in"=w319, "Part exists?"=w307, "error_in"=w320, "command_nmb"=w317) -> ("error_out"=w315:errorcluster, "user_ID"=w309:string, "save_operation_to_SQL"=w313:bool, "reference_data_to_PLC"=w318:u8[])  [unwired: 4 in]
                n95 = To Variant(anything=w318) -> (Variant=w326:variant)
                n96 = call "add_operation_to_SQL_pinion.vi"("station_number"=w312, "pinion_ID"=w308, "error_in"=w315, "user_ID"=w309, "save_operation_to_SQL"=w313, "SQL_connection_reference"=w316) -> ("error_out"=w314:errorcluster)  [unwired: 5 in]
              }
            }
          }
          frame 6 {
            # "station nmb"
            # "SAVE RESULTS"
            n97 = call-poly "byte_array_parser.vi"("error_in"=w349, "variable_start_index"=1, "byte_array"=w342) -> ("error_out"=w343:errorcluster, "U16"=w344:u16)  [unwired: 7 in]
            n98 = case shown="30" w344 {
              selector: w344 -> [w354 w413]
              tunnel: [w363 w422] -> w348
              tunnel: w347 -> [w359 w418]
              tunnel: w346 -> [w358 w417]
              tunnel: [w357 w416] -> w345
              tunnel: w343 -> [w353 w412]
              tunnel: w342 -> [w352 w411]
              tunnel: w341 -> [w351 w410]
              frame Default {
                n99 = call "get_operation_ID_from_DB.vi"("results_from_PLC"=w352, "SQL_connection_reference"=w359, "error_in"=w353, "station"=w351, "station_number"=w354) -> ("error_out"=w362:errorcluster, "operation_status"=w360:T18, "operation_ID"=w361:string, "part_ID"=w355:string)  [unwired: 3 in]
                n100 = case shown="\"PART_IN_OPERATION\"" w360 {
                  tunnel: [w368 w399 w403 w407 w409] -> w363
                  tunnel: w362 -> [w375 w399 w403 w407 w409]
                  tunnel: w361 -> [w382 _ _ _ _]
                  tunnel: w359 -> [w366 _ _ _ _]
                  tunnel: w358 -> [w387 w396 w400 w404 _]
                  tunnel: [w386 w397 w401 w405 u8[] []] -> w356
                  tunnel: w355 -> [w381 _ _ _ _]
                  tunnel: w352 -> [w372 _ _ _ _]
                  tunnel: w354 -> [w377 _ _ _ _]
                  tunnel: w351 -> [w365 _ _ _ _]
                  frame "PART_IN_OPERATION" {
                    n101 = call "get_archivisation_info_from_DB.vi"("results_from_PLC"=w372, "SQL_connection_reference"=w366, "error_in"=w375, "station"=w365, "station_number"=w377) -> ("error_out"=w371:errorcluster, "archivisation_info"=w376:string[][])  [unwired: 5 in]
                    n102 = call-poly "byte_array_parser.vi"("error_in"=w371, "variable_start_index"=53, "byte_array"=w372) -> ("error_out"=w370:errorcluster, "U8"=w373:u8)  [unwired: 7 in]
                    n103 = call "ST_parse_results_data.vi"("data_start_index"=54, "error_in"=w370, "results_from_PLC"=w372) -> ("error_out"=w378:errorcluster, "results_from_PLC"=w379:T19)  [unwired: 7 in]
                    n104 = call "prepare_inserts_for_save_results.vi"("operation_ID"=w382, "SQL_connection_reference"=w366, "error_in"=w378, "station"=w365, "results_from_PLC"=w379, "archivisation_info"=w376) -> ("error_out"=w384:errorcluster, "INSERT_statements"=w383:string[], "All PART_NUMBERS exist?"=w369:bool)  [unwired: 3 in]
                    n105 = call "append_status_updates_to_results.vi"("part_ID"=w381, "operation_ID"=w382, "opeartion_status"=w373, "error_in"=w384, "INSERT_statements"=w383) -> ("error_out"=w364:errorcluster, "INSERT_statements_with_status_updates"=w367:string[])  [unwired: 5 in]
                    n106 = case shown="True" w369 {
                      tunnel: [u8 5 ("element") u8 1 ("element")] -> w385
                      tunnel: w364 -> [w388 w394]
                      tunnel: [w388 w393] -> w368
                      tunnel: w367 -> [_ w392]
                      tunnel: w366 -> [_ w391]
                      tunnel: w365 -> [_ w390]
                      frame False {
                      }
                      frame True {
                        n107 = call "ST_do_SQL_transaction.vi"("station"=w390, "error_in"=w394, "SQL_transaction"=w392, "SQL_connection_reference"=w391) -> ("error_out"=w393:errorcluster)  [unwired: 7 in]
                      }
                    }
                    n108 = Build Array(w387, w385) -> (w386:u8[])
                  }
                  frame "PART_DOES_NOT_EXIST" {
                    n109 = Build Array(w396, u8 2 ("element")) -> (w397:u8[])
                  }
                  frame "OPERATION_DOES_NOT_EXIST" {
                    n110 = Build Array(w400, u8 3 ("element")) -> (w401:u8[])
                  }
                  frame "PART_NOT_IN_OPERATION" {
                    n111 = Build Array(w404, u8 4 ("element")) -> (w405:u8[])
                  }
                  frame Default {
                  }
                }
                n112 = To Variant(anything=w356) -> (Variant=w357:variant)
              }
              frame 30 {
                n113 = call "get_operation_ID_from_DB_pinion.vi"("results_from_PLC"=w411, "SQL_connection_reference"=w418, "error_in"=w412, "station"=w410, "station_number"=w413) -> ("error_out"=w421:errorcluster, "operation_status"=w419:T18, "operation_ID"=w420:string, "pinion_ID"=w414:string)  [unwired: 3 in]
                n114 = case shown="\"PART_IN_OPERATION\"" w419 {
                  tunnel: [w427 w458 w462 w466 w468] -> w422
                  tunnel: w421 -> [w434 w458 w462 w466 w468]
                  tunnel: w420 -> [w441 _ _ _ _]
                  tunnel: w418 -> [w425 _ _ _ _]
                  tunnel: w417 -> [w446 w455 w459 w463 _]
                  tunnel: [w445 w456 w460 w464 u8[] []] -> w415
                  tunnel: w414 -> [w440 _ _ _ _]
                  tunnel: w411 -> [w431 _ _ _ _]
                  tunnel: w413 -> [w436 _ _ _ _]
                  tunnel: w410 -> [w424 _ _ _ _]
                  frame "PART_IN_OPERATION" {
                    n115 = call "get_archivisation_info_from_DB.vi"("results_from_PLC"=w431, "SQL_connection_reference"=w425, "error_in"=w434, "station"=w424, "station_number"=w436) -> ("error_out"=w430:errorcluster, "archivisation_info"=w435:string[][])  [unwired: 5 in]
                    n116 = call-poly "byte_array_parser.vi"("error_in"=w430, "variable_start_index"=53, "byte_array"=w431) -> ("error_out"=w429:errorcluster, "U8"=w432:u8)  [unwired: 7 in]
                    n117 = call "ST_parse_results_data.vi"("data_start_index"=54, "error_in"=w429, "results_from_PLC"=w431) -> ("error_out"=w437:errorcluster, "results_from_PLC"=w438:T19)  [unwired: 7 in]
                    n118 = call "prepare_inserts_for_save_results.vi"("operation_ID"=w441, "SQL_connection_reference"=w425, "error_in"=w437, "station"=w424, "results_from_PLC"=w438, "archivisation_info"=w435) -> ("error_out"=w443:errorcluster, "INSERT_statements"=w442:string[], "All PART_NUMBERS exist?"=w428:bool)  [unwired: 3 in]
                    n119 = call "append_status_updates_to_results_pinion.vi"("pinion_ID"=w440, "operation_ID"=w441, "opeartion_status"=w432, "error_in"=w443, "INSERT_statements"=w442) -> ("error_out"=w423:errorcluster, "INSERT_statements_with_status_updates"=w426:string[])  [unwired: 5 in]
                    n120 = case shown="True" w428 {
                      tunnel: [u8 5 ("element") u8 1 ("element")] -> w444
                      tunnel: w423 -> [w447 w453]
                      tunnel: [w447 w452] -> w427
                      tunnel: w426 -> [_ w451]
                      tunnel: w425 -> [_ w450]
                      tunnel: w424 -> [_ w449]
                      frame False {
                      }
                      frame True {
                        n121 = call "ST_do_SQL_transaction.vi"("station"=w449, "error_in"=w453, "SQL_transaction"=w451, "SQL_connection_reference"=w450) -> ("error_out"=w452:errorcluster)  [unwired: 7 in]
                      }
                    }
                    n122 = Build Array(w446, w444) -> (w445:u8[])
                  }
                  frame "PART_DOES_NOT_EXIST" {
                    n123 = Build Array(w455, u8 2 ("element")) -> (w456:u8[])
                  }
                  frame "OPERATION_DOES_NOT_EXIST" {
                    n124 = Build Array(w459, u8 3 ("element")) -> (w460:u8[])
                  }
                  frame "PART_NOT_IN_OPERATION" {
                    n125 = Build Array(w463, u8 4 ("element")) -> (w464:u8[])
                  }
                  frame Default {
                  }
                }
                n126 = To Variant(anything=w415) -> (Variant=w416:variant)
              }
            }
          }
          frame 7 {
            # "station number"
            # "GET OPERATOR"
            n127 = Unbundle By Name(w487) -> ("main_ini_file.User table"=w475:string)
            n128 = call-poly "byte_array_parser.vi"("error_in"=w490, "variable_start_index"=1, "byte_array"=w486) -> ("error_out"=w478:errorcluster, "U16"=w476:u16)  [unwired: 7 in]
            n129 = call-poly "byte_array_parser.vi"("error_in"=w478, "string_length"=50, "variable_start_index"=3, "byte_array"=w486) -> ("error_out"=w474:errorcluster, "string"=w473:string)  [unwired: 6 in]
            n130 = call "Hash String with SHA-256.vi"("error_n"=w474, "string"=w473) -> ("error_out"=w470:errorcluster, "hash"=w472:string)  [unwired: 8 in]
            n131 = Format Into String(format string="SELECT  USER_NAME, ST_%d FROM %s\nWHERE BARCODE_HASH = '%s'", w476, w475, w472) -> (resulting string=w477:string)  [unwired: 2 in, 1 out]
            n132 = call "ST_do_SQL_query.vi"("station"=w471, "error_in"=w470, "SQL_query"=w477, "SQL_connection_reference"=w481) -> ("error_out"=w469:errorcluster, "recordset_out"=w479:variant[][])  [unwired: 6 in]
            n133 = call "ST_parse_operator_data.vi"("recordset_data"=w479, "error_in"=w469, "command_nmb"=w483) -> ("error_out"=w480:errorcluster, "reference_data_to_PLC"=w482:u8[])  [unwired: 7 in]
            n134 = To Variant(anything=w482) -> (Variant=w488:variant)
          }
          frame 8 {
            # "GET ST50 RESULTS"
            n135 = call-poly "byte_array_parser.vi"("error_in"=w496, "string_length"=20, "variable_start_index"=33, "byte_array"=w495) -> ("error_out"=w508:errorcluster, "string"=w507:string)  [unwired: 6 in]
            n136 = call-poly "byte_array_parser.vi"("string_length"=30, "variable_start_index"=3, "byte_array"=w495) -> ("string"=w498:string)  [unwired: 7 in, 1 out]
            n137 = call "FGV_SQL_part_ID_buffer.vi"("connection reference"=w502, "options"=FGV_SQL_part_ID_buffer."get_ID_for_name", "error_in"=w508, "station"=w492, "PART_SERIAL"=w507) -> ("error_out"=w501:errorcluster, "Part exists?"=w493:bool, "ID_out"=w494:string)  [unwired: 4 in]
            n138 = case shown="True" w493 {
              tunnel: w492 -> [_ w518]
              tunnel: [w513 w516] -> w506
              tunnel: [variant[][] [] ("recordset_out") w521] -> w505
              tunnel: w502 -> [_ w520]
              tunnel: w501 -> [w513 w517]
              tunnel: w498 -> [_ w519]
              tunnel: w494 -> [_ w515]
              frame False {
              }
              frame True {
                n139 = Format Into String(format string="EXEC GetSt50Results @ReferenceName = '%s', @PartID = %s", w519, w515) -> (resulting string=w522:string)  [unwired: 2 in, 1 out]
                n140 = call "ST_do_SQL_query.vi"("station"=w518, "error_in"=w517, "SQL_query"=w522, "SQL_connection_reference"=w520) -> ("error_out"=w516:errorcluster, "recordset_out"=w521:variant[][])  [unwired: 6 in]
              }
            }
            n141 = call "ST_parse_ST50_results_response.vi"("recordset_in"=w505, "Part exists?"=w493, "error_in"=w506, "command_nmb"=w503) -> ("error_out"=w500:errorcluster, "reference_data_to_PLC"=w504:u8[])  [unwired: 6 in]
            n142 = To Variant(anything=w504) -> (Variant=w512:variant)
          }
          frame 9 {
            # "SAVE AUDIT RESULT"
            n143 = call-poly "byte_array_parser.vi"("error_in"=w532, "variable_start_index"=1, "byte_array"=w529) -> ("error_out"=w530:errorcluster, "U16"=w531:u16)  [unwired: 7 in]
            n144 = call-poly "byte_array_parser.vi"("error_in"=w530, "variable_start_index"=3, "byte_array"=w529) -> ("error_out"=w527:errorcluster, "U8"=w528:u8)  [unwired: 7 in]
            n145 = call-poly "byte_array_parser.vi"("error_in"=w527, "string_length"=50, "variable_start_index"=4, "byte_array"=w529) -> ("error_out"=w537:errorcluster, "string"=w534:string)  [unwired: 6 in]
            n146 = Format Into String(format string="EXEC SaveAuditResult \t@StationNumber = %d, @AuditResult = %d, @UserName = '%s'", w531, w528, w534) -> (resulting string=w538:string)  [unwired: 2 in, 1 out]
            n147 = call "ST_do_SQL_query.vi"("station"=w536, "error_in"=w537, "SQL_query"=w538, "SQL_connection_reference"=w545) -> ("error_out"=w535:errorcluster, "recordset_out"=w539:variant[][])  [unwired: 6 in]
            n148 = call "ST_parse_save_audit_response.vi"("recordset_in"=w539, "error_in"=w535, "command_nmb"=w541) -> ("error_out"=w542:errorcluster, "reference_data_to_PLC"=w525:u8[])  [unwired: 7 in]
            n149 = To Variant(anything=w525) -> (Variant=w524:variant)
          }
          frame 10 {
            # "SAVE RESULTS PINION"
            n150 = call-poly "byte_array_parser.vi"("error_in"=w564, "string_length"=15, "variable_start_index"=33, "byte_array"=w552) -> ("error_out"=w563:errorcluster, "string"=w556:string)  [unwired: 6 in]
            n151 = call-poly "byte_array_parser.vi"("error_in"=w563, "variable_start_index"=48, "byte_array"=w552) -> ("error_out"=w561:errorcluster, "U8"=w562:u8)  [unwired: 7 in]
            n152 = call-poly "byte_array_parser.vi"("error_in"=w561, "string_length"=50, "variable_start_index"=49, "byte_array"=w552) -> ("error_out"=w567:errorcluster, "string"=w566:string)  [unwired: 6 in]
            n153 = Format Into String(format string="EXEC AddPinion @PinionName = '%s', @PinionStatus = %d, @UserName = '%s'", w556, w562, w566) -> (resulting string=w568:string)  [unwired: 2 in, 1 out]
            n154 = call "ST_do_SQL_query.vi"("station"=w546, "error_in"=w567, "SQL_query"=w568, "SQL_connection_reference"=w553) -> ("error_out"=w558:errorcluster, "recordset_out"=w557:variant[][])  [unwired: 6 in]
            n155 = call "ST_parse_add_pinion_response.vi"("SQL_connection_reference"=w553, "pinion_serial"=w556, "error_in"=w558, "recordset_in"=w557) -> ("error_out"=w554:errorcluster, "operation_id"=w551:string, "operation_status"=w555:T18)  [unwired: 5 in]
            n156 = case shown="\"OK\"" w555 {
              tunnel: w554 -> [w591 w597 w599]
              tunnel: [w581 w597 w599] -> w550
              tunnel: w553 -> [w576 _ _]
              tunnel: w546 -> [w588 _ _]
              tunnel: w552 -> [w585 _ _]
              tunnel: w551 -> [w582 _ _]
              tunnel: w546 -> [w573 _ _]
              tunnel: w549 -> [w579 w594 _]
              tunnel: [w578 w595 u8[] []] -> w547
              tunnel: w546 -> [w577 _ _]
              frame "OK" {
                n157 = call "get_archivisation_info_from_DB.vi"("results_from_PLC"=w585, "SQL_connection_reference"=w576, "error_in"=w591, "station"=w588, "station_number"=u16 30) -> ("error_out"=w590:errorcluster, "archivisation_info"=w583:string[][])  [unwired: 5 in]
                n158 = call "ST_parse_results_data.vi"("data_start_index"=99, "error_in"=w590, "results_from_PLC"=w585) -> ("error_out"=w589:errorcluster, "results_from_PLC"=w584:T19)  [unwired: 7 in]
                n159 = call "prepare_inserts_for_save_results.vi"("operation_ID"=w582, "SQL_connection_reference"=w576, "error_in"=w589, "station"=w577, "results_from_PLC"=w584, "archivisation_info"=w583) -> ("error_out"=w572:errorcluster, "INSERT_statements"=w580:string[], "All PART_NUMBERS exist?"=w574:bool)  [unwired: 3 in]
                n160 = call "ST_do_SQL_transaction.vi"("station"=w573, "error_in"=w572, "SQL_transaction"=w580, "SQL_connection_reference"=w576) -> ("error_out"=w581:errorcluster)  [unwired: 7 in]
                n161 = case shown="False" w574 {
                  tunnel: [u8 3 ("element") u8 1 ("element")] -> w575
                  frame False {
                  }
                  frame True {
                  }
                }
                n162 = Build Array(w579, w575) -> (w578:u8[])
              }
              frame "OPERATOR_DOES_NOT_EXIST" {
                n163 = Build Array(w594, u8 2 ("element")) -> (w595:u8[])
              }
              frame Default {
              }
            }
            n164 = To Variant(anything=w547) -> (Variant=w548:variant)
          }
          frame 11 {
            # "BIND PINION TO PART"
            n165 = call-poly "byte_array_parser.vi"("error_in"=w612, "string_length"=20, "variable_start_index"=3, "byte_array"=w611) -> ("error_out"=w607:errorcluster, "string"=w605:string)  [unwired: 6 in]
            n166 = call "FGV_SQL_part_ID_buffer.vi"("connection reference"=w602, "options"=FGV_SQL_part_ID_buffer."get_ID_for_name", "error_in"=w607, "station"=w600, "PART_SERIAL"=w605) -> ("error_out"=w606:errorcluster, "Part exists?"=w603:bool, "ID_out"=w601:string)  [unwired: 4 in]
            n167 = case shown="True" w603 {
              tunnel: [w619 w636] -> w615
              tunnel: w614 -> [w616 w635]
              tunnel: w600 -> [_ w634]
              tunnel: w611 -> [_ w633]
              tunnel: [w617 w631] -> w610
              tunnel: w606 -> [w619 w629]
              tunnel: w602 -> [_ w625]
              tunnel: w601 -> [_ w622]
              tunnel: w600 -> [_ w620]
              frame False {
                # "PART DOES NOT EXIST"
                n168 = Build Array(w616, u8 2 ("element")) -> (w617:u8[])
              }
              frame True {
                # "PART EXISTS"
                n169 = call-poly "byte_array_parser.vi"("error_in"=w629, "string_length"=15, "variable_start_index"=23, "byte_array"=w633) -> ("error_out"=w628:errorcluster, "string"=w626:string)  [unwired: 6 in]
                n170 = call "FGV_SQL_pinion_ID_buffer.vi"("connection reference"=w625, "options"=FGV_SQL_pinion_ID_buffer."get_ID_for_name", "error_in"=w628, "station"=w620, "PINION_SERIAL"=w626) -> ("error_out"=w623:errorcluster, "Pinion exists?"=w624:bool, "ID_out"=w621:string)  [unwired: 4 in]
                n171 = case shown="True" w624 {
                  tunnel: [w640 w652] -> w636
                  tunnel: w635 -> [w637 w649]
                  tunnel: w634 -> [_ w654]
                  tunnel: [w638 w650] -> w631
                  tunnel: w625 -> [_ w647]
                  tunnel: w623 -> [w640 w653]
                  tunnel: w622 -> [_ w645]
                  tunnel: w621 -> [_ w646]
                  frame False {
                    # "PINION DOES NOT EXIST"
                    n172 = Build Array(w637, u8 3 ("element")) -> (w638:u8[])
                  }
                  frame True {
                    # "PINION EXISTS"
                    n173 = Format Into String(format string="UPDATE PRODUCTION_PARTS SET\nPINION_ID = %s WHERE ID = %s;", w646, w645) -> (resulting string=w642:string)  [unwired: 2 in, 1 out]
                    n174 = Format Into String(format string="UPDATE PRODUCTION_PINIONS SET\nPART_ID = %s WHERE ID = %s;", w645, w646) -> (resulting string=w641:string)  [unwired: 2 in, 1 out]
                    n175 = Build Array(w642, w641) -> (w643:string[])
                    n176 = call "ST_do_SQL_transaction.vi"("station"=w654, "error_in"=w653, "SQL_transaction"=w643, "SQL_connection_reference"=w647) -> ("error_out"=w652:errorcluster)  [unwired: 7 in]
                    n177 = Build Array(w649, u8 1 ("element")) -> (w650:u8[])
                  }
                }
              }
            }
            n178 = To Variant(anything=w610) -> (Variant=w609:variant)
          }
          frame Default {
            # "UNKNOWN COMMAND"
            n179 = call-poly "Get Localized Phrase Compact Interface.vi"("Key"="Unknown command from PLC received. Command: %d" ("source")) -> ("Translated Phrase"=w655:string)
            n180 = Format Into String(format string=w655, w658) -> (resulting string=w657:string)  [unwired: 2 in, 1 out]
            n181 = Bundle By Name(cluster=errorcluster {"status"=TRUE, "code"=500, "source"=""} ("error_out"), "source"=w657) -> (w656:errorcluster)
          }
        }
        n182 = call "ST_SQL_check_for_error.vi"("ST_SQL_loop_state_in"=ST_SQL_sequence_state."send_to_PLC" ("ST_MAIN_sequence_state"), "error_in"=w165) -> ("ST_SQL_loop_state_out"=w171:T6, "error_out"=w173:errorcluster)  [unwired: 8 in]
      }
      frame "send_to_PLC" {
        n183 = Variant To Data(error in=w668, type=u8[] [], Variant=w669) -> (data=w663:u8[], error out=w662:errorcluster)
        n184 = call "FGV_PROXY_connection_references.vi"("station"=w666, "options"=FGV_PROXY_connection_references."get", "error_in"=w662) -> ("error_out"=w672:errorcluster, "connection_ID_out"=w671:refnum<k5>)  [unwired: 5 in, 2 out]
        n185 = TCP Write(connection ID=w671, data in=w663, error in (no error)=w672) -> (error out=w665:errorcluster)  [unwired: 1 in, 2 out]
        n186 = Byte Array To String(unsigned byte array=w663) -> (string=w661:string)
        n187 = case shown="No Error" w665 {
          selector: w665 -> [w681 w683]
          tunnel: w666 -> [w682 _]
          tunnel: [w680 w683] -> w664
          tunnel: w661 -> [w679 _]
          frame No Error {
            n188 = To Variant(anything=w679) -> (Variant=w677:variant)
            n189 = call "FGV_PROXY_DIAGNOSTICS_message_history_buffer.vi"("station"=w682, "options"=FGV_PROXY_DIAGNOSTICS_message_history_buffer."add_TCP_PC_to_PLC", "error_in"=w681, "input"=w677) -> ("error_out"=w680:errorcluster)  [unwired: 6 in, 1 out]
          }
          frame Error {
          }
        }
        n190 = call "ST_SQL_check_for_error.vi"("ST_SQL_loop_state_in"=ST_SQL_sequence_state."get_next_state" ("PLC_MAIN_loop_state_in"), "error_in"=w664) -> ("ST_SQL_loop_state_out"=w675:T6, "error_out"=w676:errorcluster)  [unwired: 8 in]
      }
      frame "error" {
        w690 = T17 refnum items=["Connection"] ("connection reference")
        n191 = To Variant(anything=PROXY_SQL_connection_status."Error" ("SQL_connection_status")) -> (Variant=w686:variant)
        n192 = call "FGV_PROXY_DIAGNOSTICS_records_display.vi"("options"=FGV_PROXY_DIAGNOSTICS_records_display."set_SQL_connection_status", "error_in"=w688, "station"=w684, "input"=w686) -> ("error_out"=w687:errorcluster)  [unwired: 6 in, 1 out]
        n193 = call "FGV_PROXY_error_buffer.vi"("station"=w684, "option"=FGV_PROXY_error_buffer."display", "error_in"=w687) -> ("error_out"=w692:errorcluster)  [unwired: 7 in, 1 out]
        n194 = call <vilib>:"DB Tools Close Connection.vi"("error in (no error)"=w692, "connection reference"=w693) -> ("error out"=w691:errorcluster)  [unwired: 5 in]
        n195 = call "ST_SQL_check_for_error.vi"("ST_SQL_loop_state_in"=ST_SQL_sequence_state."initialize" ("ST_MAIN_sequence_state"), "error_in"=w691) -> ("ST_SQL_loop_state_out"=w694:T6, "error_out"=w697:errorcluster)  [unwired: 8 in]
        n196 = call "wait_on_initialization.vi"("state"=w694) -> ()  [unwired: 11 in]
      }
      frame "stop" {
        w700 = T17 refnum items=["Connection"] ("connection reference")
        n197 = call <vilib>:"Clear Errors.vi"("error in (no error)"=w699) -> ("error out"=w698:errorcluster)  [unwired: 5 in, 1 out]
        n198 = call <vilib>:"DB Tools Close Connection.vi"("error in (no error)"=w698, "connection reference"=w701) -> ("error out"=w703:errorcluster)  [unwired: 5 in]
      }
    }
  }
  n199 = Merge Errors(w6, w7) -> (→"error_out":errorcluster)
